vi "CSDB_Transfer.get all instances from DB.vi"(4 "error in (no error)":errorcluster, 7 "Data Source":string) -> (0 "error out":errorcluster, 3 "sorted array":string[](array[string]))   [LabVIEW 2014, in "CSDB_Transfer.lvlib"]
doc: "Open a connection to the database and reads all instancenames. The connection is closed afterwards."
uses:
  CSDB_Transfer.lvlib
  <vilib>/addons/database/Connection.llb/DB Tools Open Connec (String).vi
  <vilib>/addons/database/NI_Database_API.lvlib
  CSDB_Common/CSDB_Common.lvlib
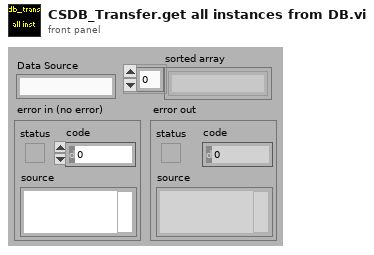
[diagram p1: front panel]
types:
  T1 = typedef "NI_Database_API.lvlib/Conn ObjectReference.ctl" = refnum<k1>
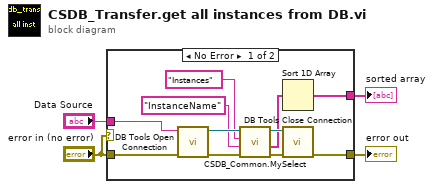
[diagram p0: block diagram]
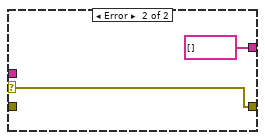
[diagram p2: hidden frame]
diagram:
  n1 = case shown="No Error" "error in (no error)" {
    selector: "error in (no error)" -> [_ w17]
    tunnel: [w9 w17] -> w4
    tunnel: "Data Source" -> [w7 _]
    tunnel: "error in (no error)" -> [w6 _]
    tunnel: [w5 string[] []] -> w2
    frame No Error {
      n2 = call-poly <vilib>:"DB Tools Open Connection.vi"("error in (no error)"=w6, "connection information"=w7) -> ("error out"=w14:errorcluster, "connection reference"=w15:T1)  [unwired: 6 in]
      n3 = call "CSDB_Common.MySelect.vi"("error in (no error)"=w14, "column"="InstanceName", "table"="Instances", "connection reference"=w15) -> ("error out"=w10:errorcluster, "1d output array"=w8:string[], "connection reference out"=w11:T1)  [unwired: 3 in]
      n4 = Sort 1D Array(array=w8) -> (sorted array=w5:string[])
      n5 = call <vilib>:"DB Tools Close Connection.vi"("error in (no error)"=w10, "connection reference"=w11) -> ("error out"=w9:errorcluster)  [unwired: 5 in]
    }
    frame Error {
    }
  }
  "error out" <- w4
  "sorted array" <- w2
